vi "Data Column Names.vi"(4 "error in":errorcluster) -> (0 "error out":errorcluster, 3 "Array":string[](array[string]))   [LabVIEW 2023]
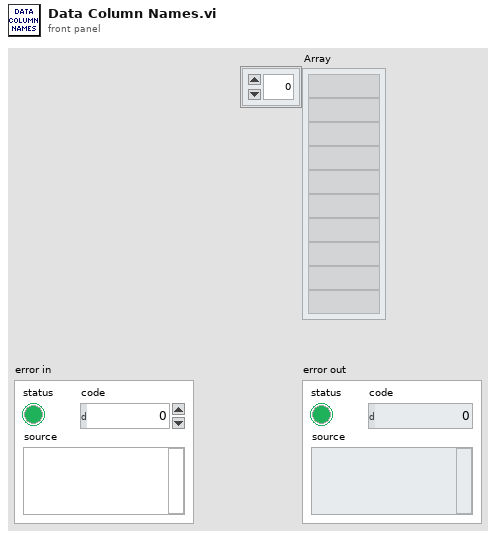
[diagram p1: front panel]
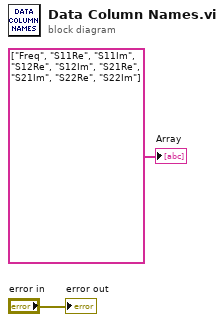
[diagram p0: block diagram]
diagram:
  "Array" <- string[] ["Freq", "S11Re", "S11Im", "S12Re", "S12Im", "S21Re", "S21Im", "S22Re", "S22Im"]
  "error out" <- "error in"
